vi "Error Report Informations.vi"() -> (0 "Error Descriptions Out":string[](array[string])=["", "You have no right to access the output folder.", "Please input a valid library name.", "Please contact National Instruments for help.", "Bad value was passed into a function (e.g. empty file name).", "Possible Reasons are:\n1. The URL does not exist or the WSDL is bad.\n2. Authentication is not correct.\n3. Proxy information is not correct.", "Validation failed. The URL is not formatted correctly and should be in the following form: http://localhost/test/good.asmx?WSDL", "Bad host name. (e.g. http://local host/test/test.asmx)", "LabVIEW is unable to create a directory for the imported DLL.", "Possible reasons are:\n1. The output file(s) might be read-only.\n     Remove the read-only attribute and import the Web service again.\n2.  A proxy DLL that LabVIEW created under the same file path exists in memory.\n     Restart LabVIEW and import the Web service again.", "Possible Reasons are:\n1.\tThe VI under the specified path is write-protected. \n   Remove the write-protected attribute and import the web service again.\n2.\tA VI with the same name exists in memory.\n   Close the VI and import the web service again to overwirte it.\n3.\tThe web service method that you use to create the wrapper VI has more than 12 parameters. \n   Complete the following steps to resolve this error.\n   1) Open LabVIEW and open the LabVIEW library file.  \n   2)\tIn the imported VIs folder, duplicate one of the VIs and rename it.\n   3)\tAdd the new VI to the LabVIEW library file.\n   4)\tOpen the front panel of the VI and change the connector pane to use a pattern with more inputs. For example, 6-2-2-2-2-6. Verify that the refnums and error inputs are assigned to the corners of the connector pane.\n   5) Open the block diagram of the VI and change the invoke node to the method you want to import. Do not select either of the asynchronous Begin... or End... messages, they do not work in LabVIEW 8.2.\n   6)\tDelete the obsolete controls and indicators, if any.\n   7)\tFor each of the inputs and outputs of the method, create an indicator or control.\n   8)\tOn the front panel, assign the new controls and indicators to the connector pane.\n   9)\tArrange the controls and indicators appropriately.\n   10)\tSave the VI and the LabVIEW library file. ", "Project Library Generation Failed.\nPossible Reasons:\n1. The imported project library has a conflicting name with a project library already in memory.\n2. The imported VIs have conflicting names with VIs already in memory.\nClose the project library and VIs and reimport the Web Service.  ", "Error message from C# compiler:"], 1 "Error Titles Out":string[](array[string])=["No Error.", "Unauthorized Access.", "Invalid Library Name.", "Internal Unknown Error.", "WSDL Validation Failed.", "Validation Failed.", "WSDL Validation Failed.", "WSDL Validation Failed.", "Can't create local proxy dll.", "Can't generate files.", "Can't Create Wrapper VIs.", "Can't Create Project Library.", "Cannot generate C# assembly."], 2 "Error Numbers Out":T1[](array[typedef])=[0, 1, 2, 201, 202, 203, 204, 205, 206, 207, 3, 208, 209] items=["ERR_NOERROR"=0, "ERR_ACCESS_OUTPUTFOLDER"=1, "ERR_INVALID_LIBRARYNAME"=2, "ERR_CREATE_VIWRAPPER"=3, "ERR_UNKNOWN"=201, "ERR_BAD_ARGUMENT"=202, "ERR_URL_NOTFOUND_BADWSDL"=203, "ERR_BADLYFORMATTEDURL"=204, "ERR_BADHOSTNAME"=205, "ERR_BADDIRECTORY"=206, "ERR_UNAUTHORIZEDACCESS"=207, "ERR_CREATELIBRARY"=208, "ERR_COMPILEERROR"=209])   [LabVIEW 2017, in "WebServiceImporter.lvlib" / "Error Handling.lvlib"]
uses:
  <vilib>/Platform/WebService/Error Handling/Error Handling.lvlib
  <vilib>/Platform/WebService/Error Handling/Error/Error Number.ctl
panel:
  in  "Error Descriptions Constant":string[](array[string])=["", "You have no right to access the output folder.", "Please input a valid library name.", "Please contact National Instruments for help.", "Bad value was passed into a function (e.g. empty file name).", "Possible Reasons are:\n1. The URL does not exist or the WSDL is bad.\n2. Authentication is not correct.\n3. Proxy information is not correct.", "Validation failed. The URL is not formatted correctly and should be in the following form: http://localhost/test/good.asmx?WSDL", "Bad host name. (e.g. http://local host/test/test.asmx)", "LabVIEW is unable to create a directory for the imported DLL.", "Possible reasons are:\n1. The output file(s) might be read-only.\n     Remove the read-only attribute and import the Web service again.\n2.  A proxy DLL that LabVIEW created under the same file path exists in memory.\n     Restart LabVIEW and import the Web service again.", "Possible Reasons are:\n1.\tThe VI under the specified path is write-protected. \nSolution: remove the write-protected attribute and import the web service again.\n2.\tA VI with the same name exists in memory.\nSolution: close the VI and import the web service again to overwirte it.\n3.\tThe web service method that you use to create the wrapper VI has more than 12 parameters. \nSolution: follow the steps to manually create wrapper VI with more than 12 parameters.\n   1) Open LabVIEW and open the LabVIEW library file.  \n   2)\tIn the imported VIs folder, duplicate one of the VIs and rename it.\n   3)\tAdd the new VI to the LabVIEW library file.\n   4)\tOpen the front panel of the VI and change the connector pane to use a pattern with more inputs. For example, 6-2-2-2-2-6. Verify that the refnums and error inputs are assigned to the corners of the connector pane.\n   5) Open the block diagram of the VI and change the invoke node to the method you want to import. Do not select the asynchronous methods named by Begin... or End... since they do not work in LabVIEW.\n   6)\tDelete the obsolete controls and indicators, if any.\n   7)\tFor each of the inputs and outputs of the method, create an indicator or control.\n   8)\tOn the front panel, assign the new controls and indicators to the connector pane.\n   9)\tArrange the controls and indicators appropriately.\n   10)\tSave the VI and the LabVIEW library file. ", "Project Library Generation Failed.\nPossible Reasons:\n1. The imported project library has a conflicting name with a project library already in memory.\n2. The imported VIs have conflicting names with VIs already in memory.\nClose the project library and VIs and reimport the Web Service.  ", "Error message from C# compiler:"]
  in  "Error Titles Constant":string[](array[string])=["No Error.", "Unauthorized Access.", "Invalid Library Name.", "Internal Unknown Error.", "WSDL Validation Failed.", "Validation Failed.", "WSDL Validation Failed.", "WSDL Validation Failed.", "Can't create local proxy dll.", "Can't generate files.", "Can't Create Wrapper VIs for Following Web Methods.", "Can't Create Project Library.", "Cannot generate C# assembly."]
  in  "Error Numbers Constant":T1[](array[typedef])=[0, 1, 2, 201, 202, 203, 204, 205, 206, 207, 3, 208, 209] items=["ERR_NOERROR"=0, "ERR_ACCESS_OUTPUTFOLDER"=1, "ERR_INVALID_LIBRARYNAME"=2, "ERR_CREATE_VIWRAPPER"=3, "ERR_UNKNOWN"=201, "ERR_BAD_ARGUMENT"=202, "ERR_URL_NOTFOUND_BADWSDL"=203, "ERR_BADLYFORMATTEDURL"=204, "ERR_BADHOSTNAME"=205, "ERR_BADDIRECTORY"=206, "ERR_UNAUTHORIZEDACCESS"=207, "ERR_CREATELIBRARY"=208, "ERR_COMPILEERROR"=209]
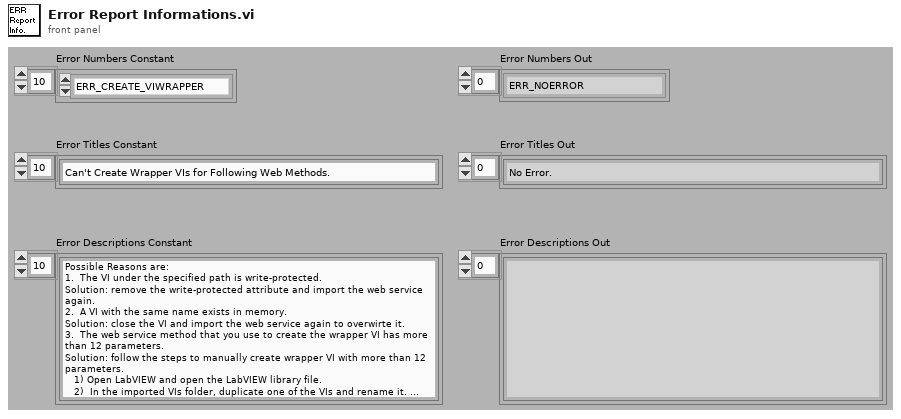
[diagram p1: front panel]
types:
  T1 = typedef "WebServiceImporter.lvlib/Error Handling.lvlib/Error Number.ctl" = u16
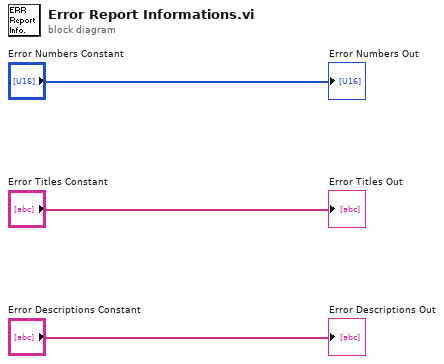
[diagram p0: block diagram]
diagram:
  "Error Numbers Out" <- "Error Numbers Constant"
  "Error Titles Out" <- "Error Titles Constant"
  "Error Descriptions Out" <- "Error Descriptions Constant"
